vi "Alarme.vi"(8 "alarme":bool, 9 "seuil bas":dbl=69.0, 10 "seuil haut":dbl=71.0, 11 "fréquence cardiaque":dbl) -> (3 "Alerte visuelle":bool)   [LabVIEW 2017]
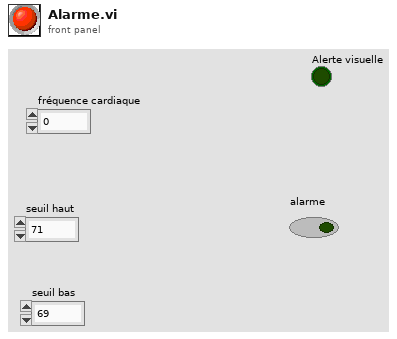
[diagram p1: front panel]
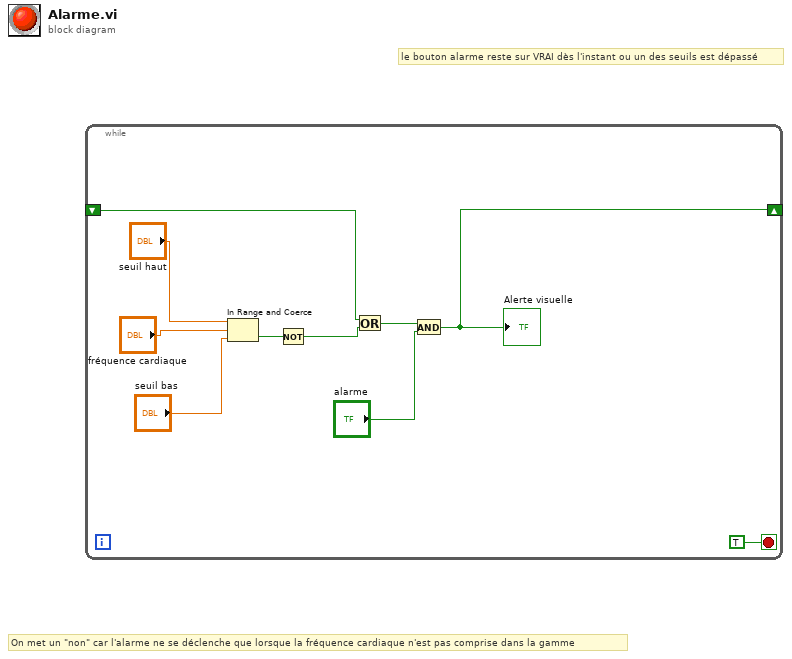
[diagram p0: block diagram]
diagram:
  # "le bouton alarme reste sur VRAI dès l'instant ou un des seuils est dépassé"
  # "On met un \"non\" car l'alarme ne se déclenche que lorsque la fréquence cardiaque n'est pas comprise dans la gamme"
  n1 = while {
    shift-right: [w1] -> _
    shift-left: _ -> [w4]
    stop <- TRUE stop-if-true
    n2 = In Range and Coerce(upper limit="seuil haut", x="fréquence cardiaque", lower limit="seuil bas") -> (In Range?=w7:bool)  [unwired: 1 out]
    n3 = Not(x=w7) -> (.not. x?=w5:bool)
    n4 = Or(x=w4, y=w5) -> (x .or. y?=w3:bool)
    n5 = And(x=w3, y="alarme") -> (x .and. y?=w1:bool)
    "Alerte visuelle" <- w1
  }
